vi "serviceMode_disable.vi"(8 "error in (no error)":errorcluster, 11 "Thorlabs_OSA300_64 in":refnum<class "OSA300.lvclass">) -> (0 "error out":errorcluster, 3 "Thorlabs_OSA300_64 out":refnum<class "OSA300.lvclass">)   [LabVIEW 2010, in "OSA300.lvclass"]
uses:
  OSA300.lvclass
  FTSLib.dll
  OSA.lvclass
  OSA20X_misc.lvlib
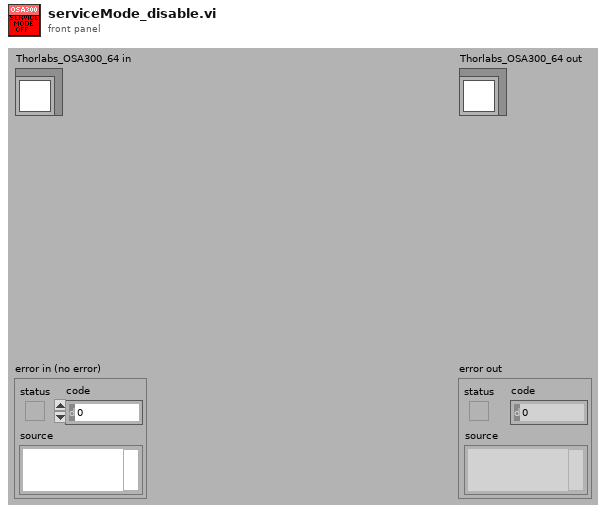
[diagram p1: front panel]
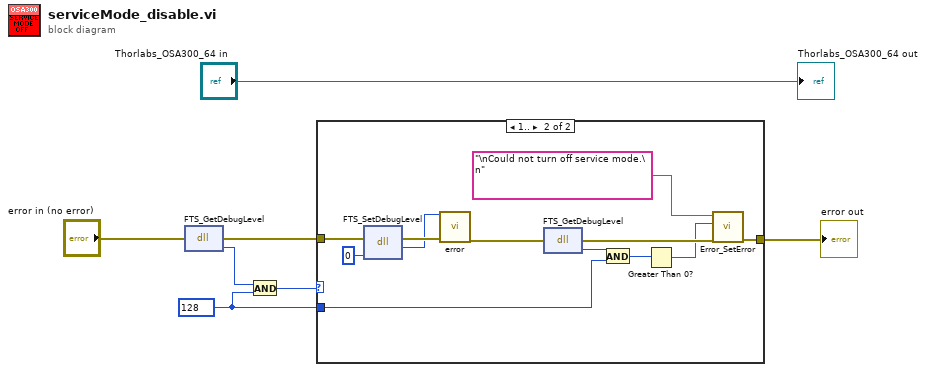
[diagram p0: block diagram]
diagram:
  w1 = u16 128 ("debugLevel")
  n1 = dll-call lib="FTSLib.dll" fn="FTS_GetDebugLevel"(error in="error in (no error)") -> (error out=w3:errorcluster, "return type"=w4:u16)  [unwired: 2 in, 1 out]
  n2 = And(x=w4, y=w1) -> (x .and. y?=w2:u16)
  n3 = case shown="1.." w2 {
    tunnel: [w8 w11] -> w6
    tunnel: w3 -> [w8 w10]
    tunnel: w1 -> [_ w9]
    frame 0, Default {
    }
    frame 1.. {
      n4 = dll-call lib="FTSLib.dll" fn="FTS_SetDebugLevel"(error in=w10, "debugLevel"=u16 0) -> (error out=w19:errorcluster, "return type"=w18:i32)  [unwired: 3 in, 1 out]
      n5 = call "error.vi"("result code"=w18, "error in (no error)"=w19) -> ("error out"=w17:errorcluster)  [unwired: 15 in, 2 out]
      n6 = dll-call lib="FTSLib.dll" fn="FTS_GetDebugLevel"(error in=w17) -> (error out=w14:errorcluster, "return type"=w16:u16)  [unwired: 2 in, 1 out]
      n7 = And(x=w16, y=w9) -> (x .and. y?=w15:u16)
      n8 = Greater Than 0?(x=w15) -> (x > 0?=w13:bool)
      n9 = call "Error_SetError.vi"("error in"=w14, "status (true)"=w13, "source(\"\")"="\nCould not turn off service mode.\n" ("source(\"\")")) -> ("error out"=w11:errorcluster)  [unwired: 4 in]
    }
  }
  "error out" <- w6
  "Thorlabs_OSA300_64 out" <- "Thorlabs_OSA300_64 in"
